vi "dfd_Nyquist Filter Design TF Modify.vi"(9 "band":i32, 11 "tf":dbl[](array[numeric])) -> (3 "new tf":dbl[](array[numeric]))   [LabVIEW 2017, in "NI_DigFilter_Process.lvlib"]
uses:
  <vilib>/addons/Digital Filter Design/NI_DigFilter_Process.lvlib
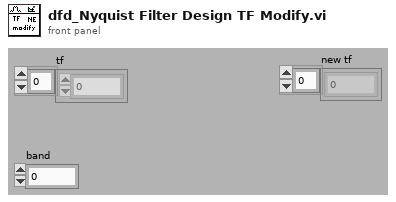
[diagram p1: front panel]
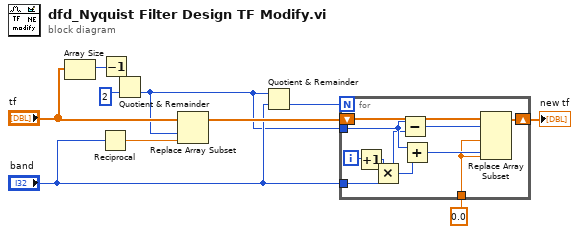
[diagram p0: block diagram]
diagram:
  n1 = Array Size(array="tf") -> (size(s)=w7:i32)
  n2 = Reciprocal(x="band") -> (1/x=w1:dbl)
  n3 = Decrement(x=w7) -> (x-1=w6:i32)
  n4 = Quotient & Remainder(x=w6, y=2) -> (floor(x/y)=w2:i32)  [unwired: 1 out]
  n5 = Replace Array Subset(array="tf", new element=w1, index=w2) -> (w4:dbl[])
  n6 = Quotient & Remainder(x=w2, y="band") -> (floor(x/y)=w9:i32)  [unwired: 1 out]
  n7 = for {
    N: w9 -> [_]
    tunnel: w2 -> [w18]
    tunnel: "band" -> [w20]
    shift-right: [w14] -> w10
    shift-left: w4 -> [w21]
    tunnel: 0.0 -> [w12]
    i -> [w19]
    n8 = Increment(x=w19) -> (x+1=w13:i32)
    n9 = Multiply(x=w13, y=w20) -> (x*y=w17:i32)
    n10 = Subtract(x=w18, y=w17) -> (x-y=w16:i32)
    n11 = Add(x=w18, y=w17) -> (x+y=w15:i32)
    n12 = Replace Array Subset(array=w21, new element #1=w12, index #1=w16, new element #2=w12, index #2=w15) -> (w14:dbl[])
  }
  "new tf" <- w10
